vi "smartmeshIP get data packet.vi"(6 "use correction":bool=TRUE, 8 "error in":errorcluster, 10 "commandType":u8, 11 "data":string) -> (0 "error out":errorcluster, 2 "mote and link status":T2, 3 "Data Notifications":T3)   [LabVIEW 2017]
panel:
  out "network time":T1
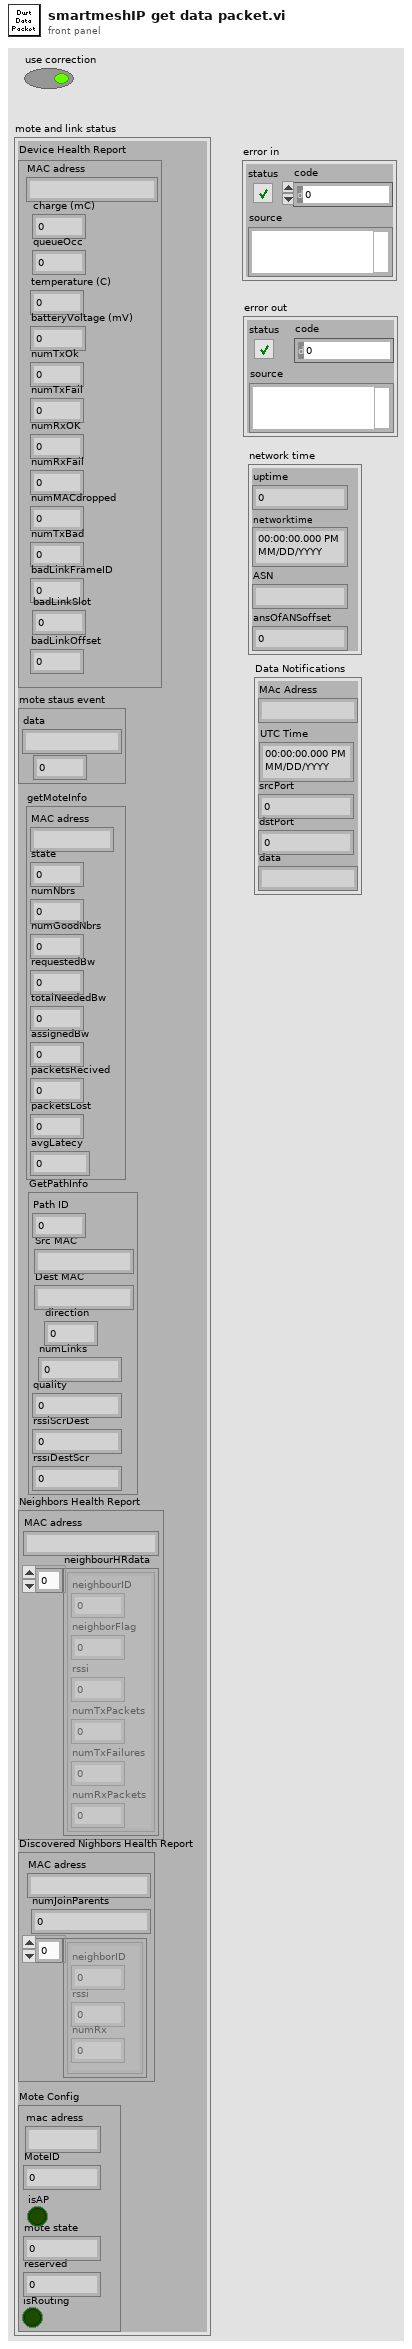
[diagram p1: front panel]
types:
  T1 = cluster{"uptime":u32, "networktime":timestamp, "ASN":string, "ansOfANSoffset":u16}
  T2 = cluster{"Device Health Report":cluster{"MAC adress":string, "charge (mC)":u32, "queueOcc":u8, "temperature (C)":i8, "batteryVoltage (mV)":u16, "numTxOk":u16, "numTxFail":u16, "numRxOK":u16, "numRxFail":u16, "numMACdropped":u8, "numTxBad":u8, "badLinkFrameID":u8, "badLinkSlot":u32, "badLinkOffset":u8}, "mote staus event":cluster{"data":string, u8}, "getMoteInfo":cluster{"MAC adress":string, "state":u8, "numNbrs":u8, "numGoodNbrs":u8, "requestedBw":u32, "totalNeededBw":u32, "assignedBw":u32, "packetsRecived":u32, "packetsLost":u32, "avgLatecy":u32}, "GetPathInfo":cluster{"Path ID":u8, "Src MAC":string, "Dest MAC":string, "direction":u8, "numLinks":u8, "quality":u8, "rssiScrDest":i8, "rssiDestScr":i8}, "Neighbors Health Report":cluster{"MAC adress":string, "neighbourHRdata":cluster{"neighbourID":u16, "neighborFlag":u8, "rssi":i8, "numTxPackets":u16, "numTxFailures":u16, "numRxPackets":u16}[]}, "Discovered Nighbors Health Report":cluster{"MAC adress":string, "numJoinParents":u8, cluster{"neighborID":u16, "rssi":i8, "numRx":u8}[]}, "Mote Config":cluster{"mac adress":string, "MoteID":u16, "isAP":bool, "mote state":u8, "reserved":u8, "isRouting":bool}}
  T3 = cluster{"MAc Adress":string, "UTC Time":timestamp, "srcPort":u16, "dstPort":u16, "data":string}
  T4 = cluster{"index":u32, "Dust Timestamp":timestamp, "data":string, "index":u16}
  T5 = cluster{"data":string, "Dust Timestamp":timestamp, u16, u16, "data":string}
  T6 = cluster{"data":string, u32, u8, i8, u16, u16, u16, u16, u16, u8, u8, u8, u32, u8}
  T7 = cluster{"data":string, cluster{u16, u8, i8, u16, u16, u16}[]}
  T8 = cluster{"data":string, u8, cluster{u16, i8, u8}[]}
  T9 = cluster{"(hi.lo)":u16, "data":string, "data":string, u8, u8, u8, i8, i8}
  T10 = cluster{u16, "data":string, "data":string, u8, u8, u8, i8, i8}
  T11 = cluster{"data":string, u8, u8, u8, u32, u32, u32, u32, u32, u32}
  T12 = cluster{cluster{"data":string, u32, u8, i8, u16, u16, u16, u16, u16, u8, u8, u8, u32, u8}, cluster{"data":string, i32}, cluster{"data":string, u8, u8, u8, u32, u32, u32, u32, u32, u32}, cluster{"(hi.lo)":u16, "data":string, "data":string, u8, u8, u8, i8, i8}, cluster{"data":string, cluster{u16, u8, i8, u16, u16, u16}[]}, cluster{"data":string, u8, cluster{u16, i8, u8}[]}, cluster{"data":string, u16, bool, u8, u8, bool}}
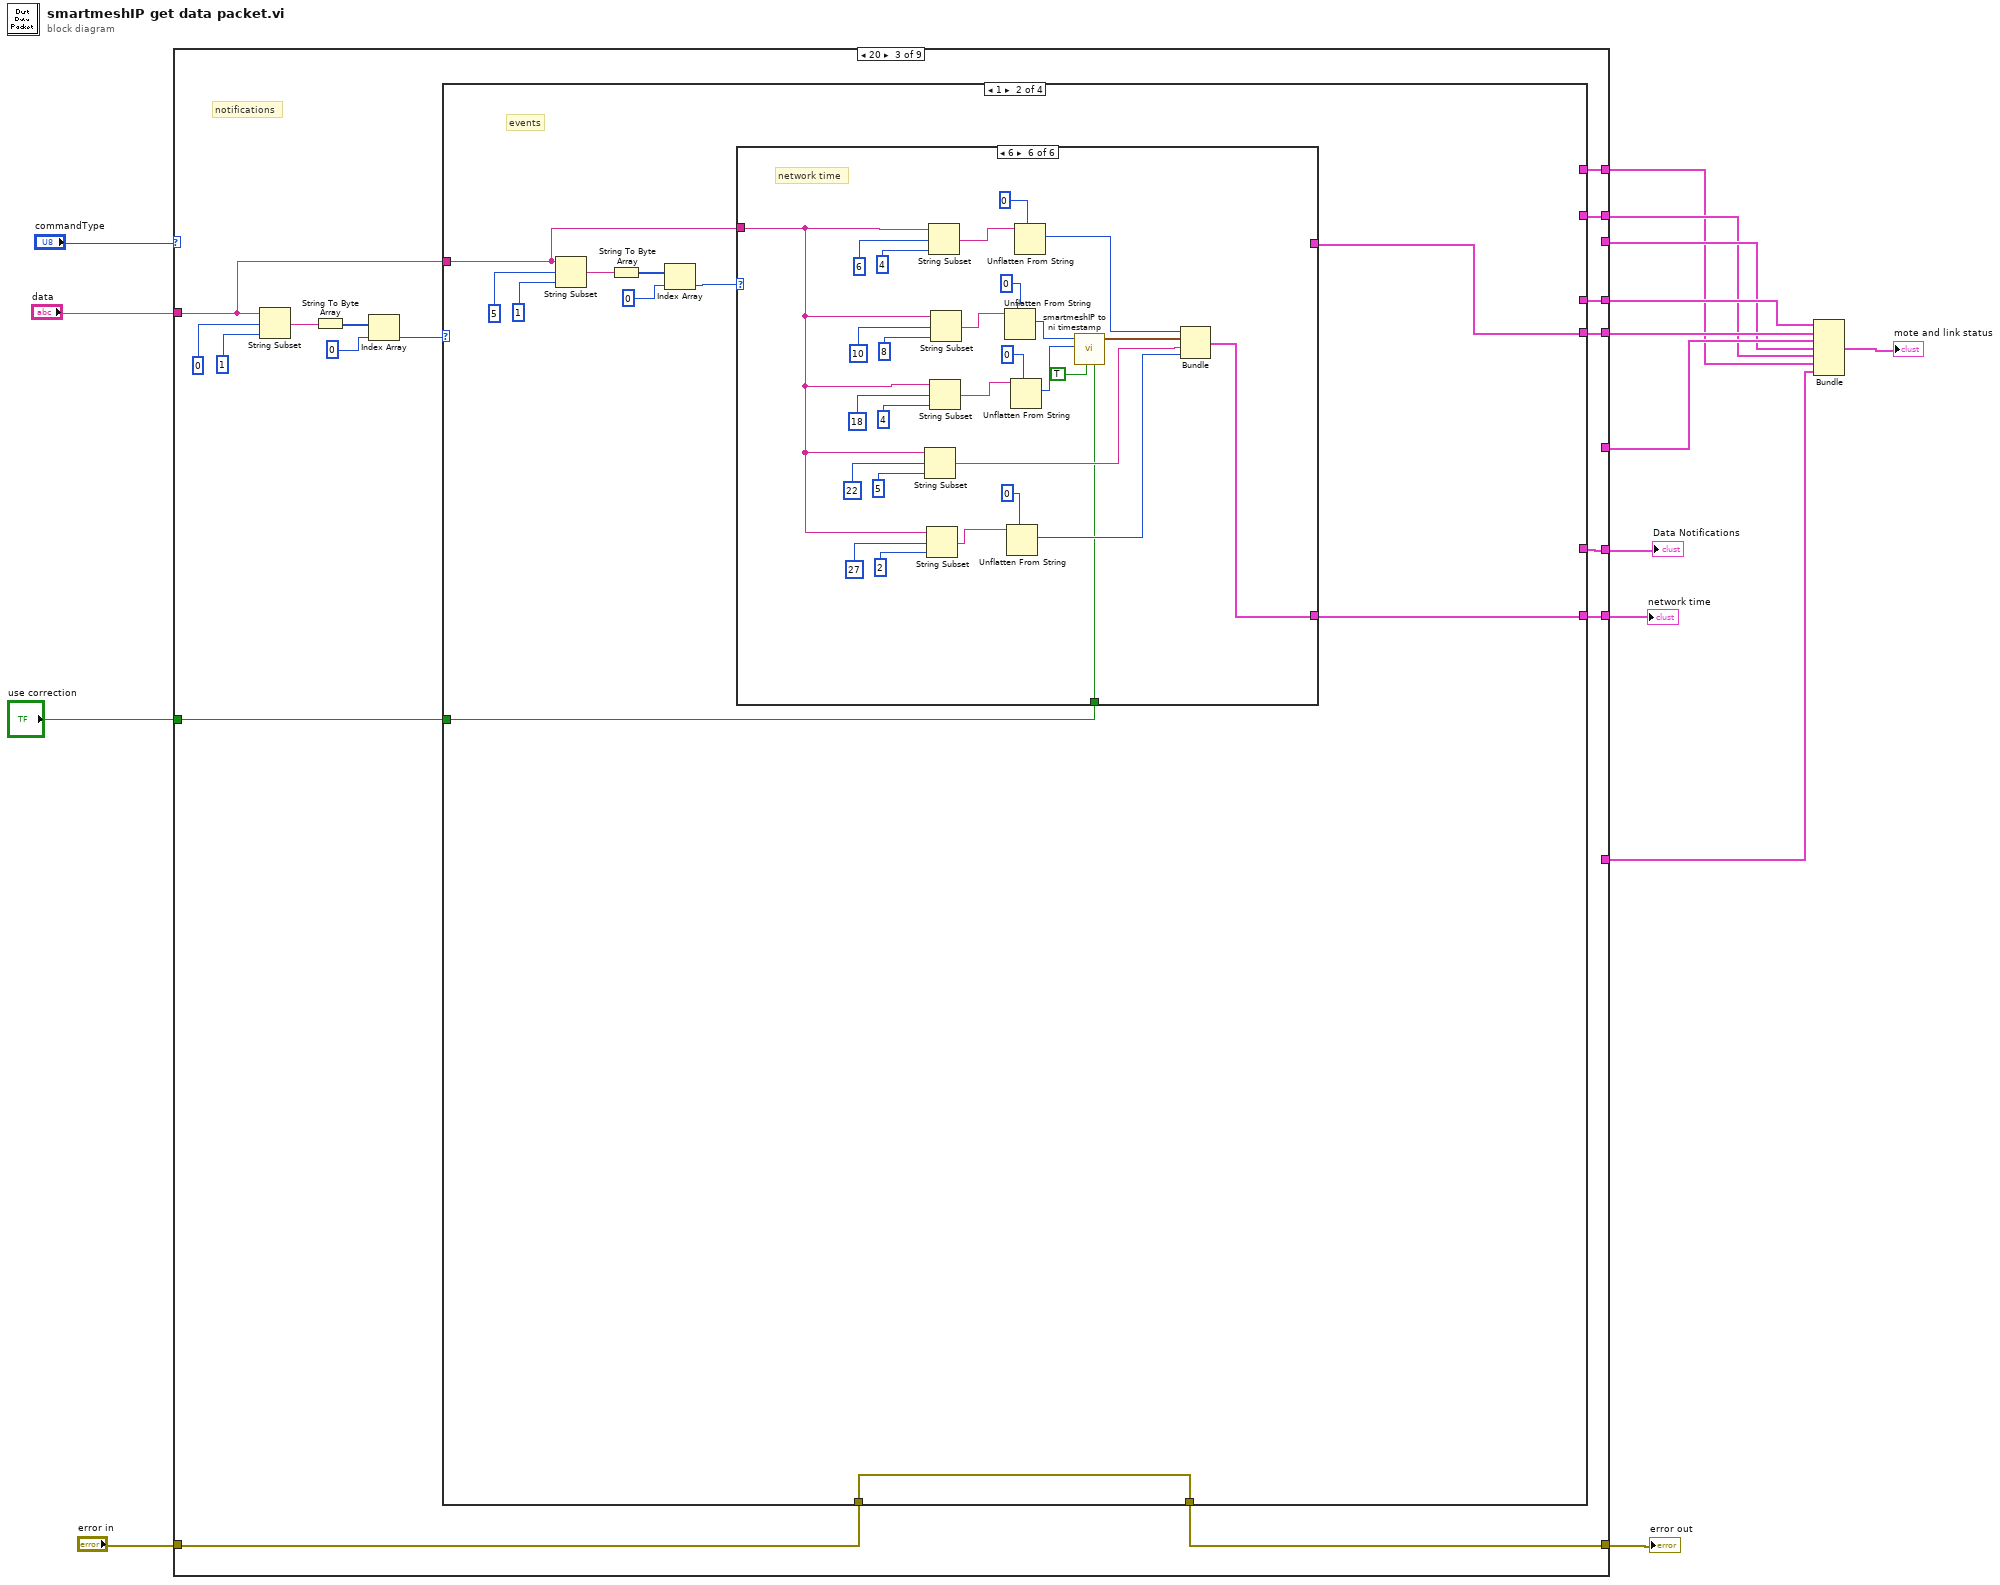
[diagram p0: block diagram]
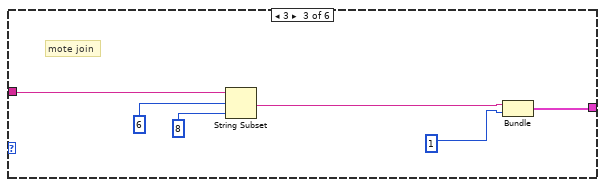
[diagram p7: hidden frame]
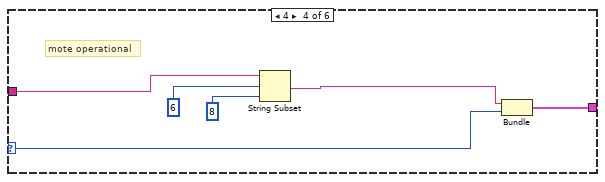
[diagram p8: hidden frame]
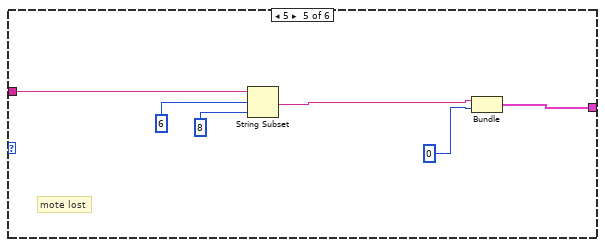
[diagram p9: hidden frame]
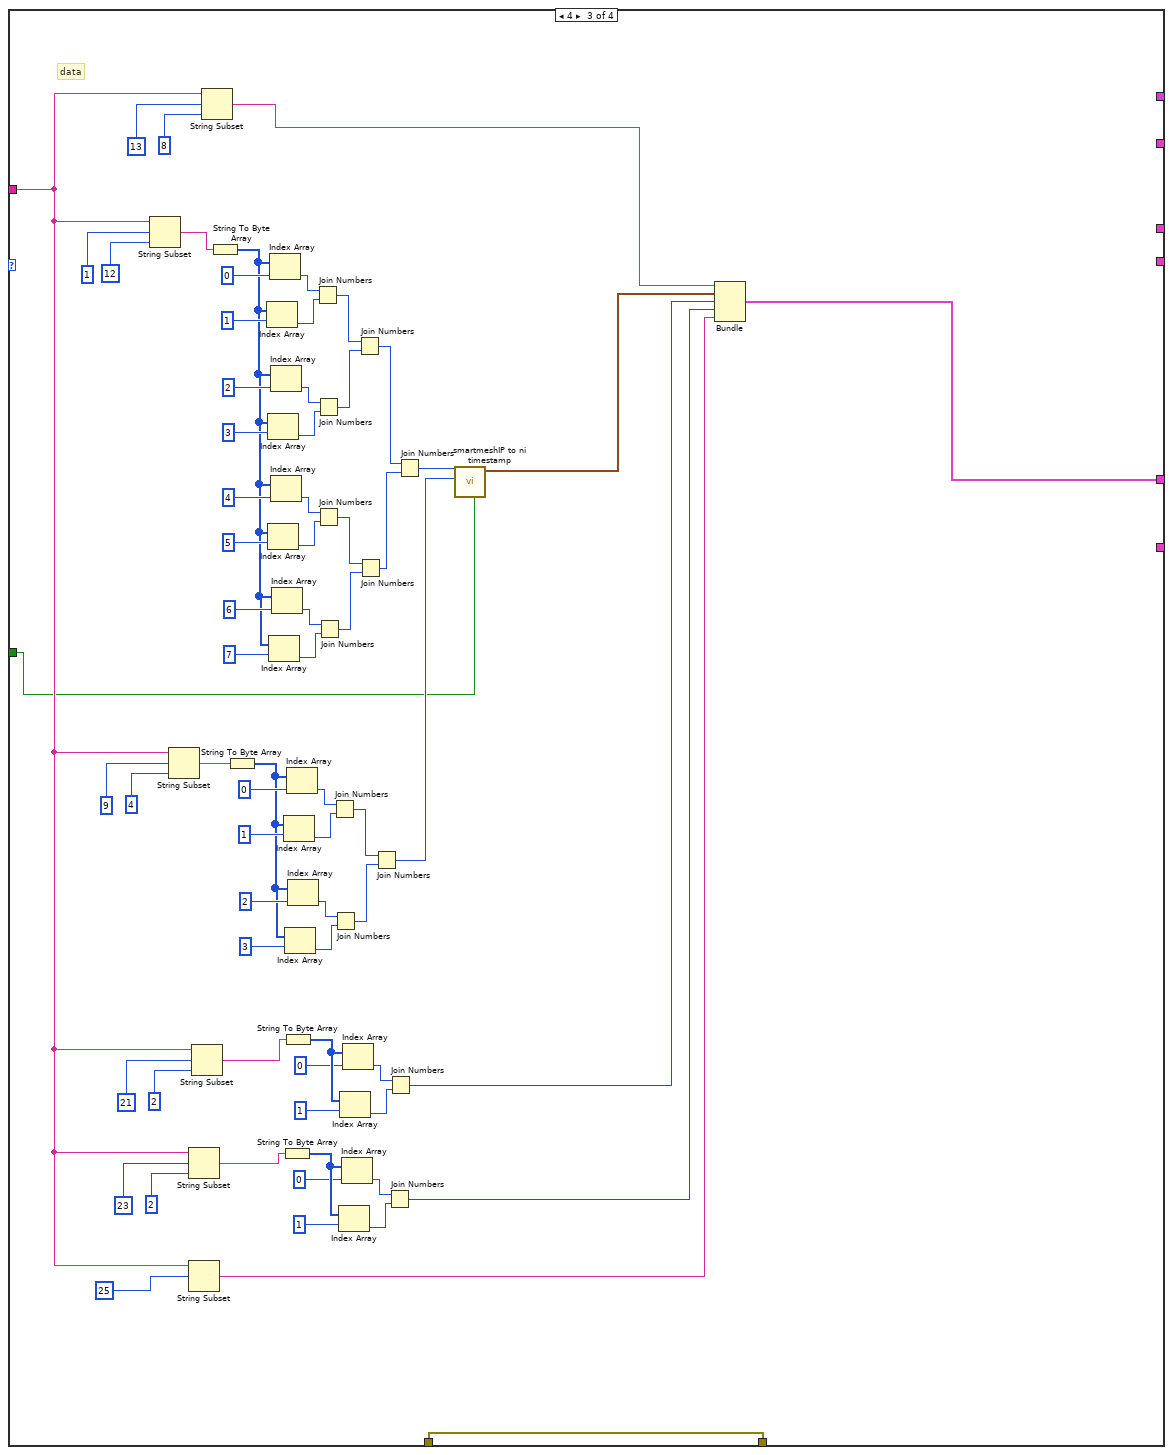
[diagram p10: hidden frame]
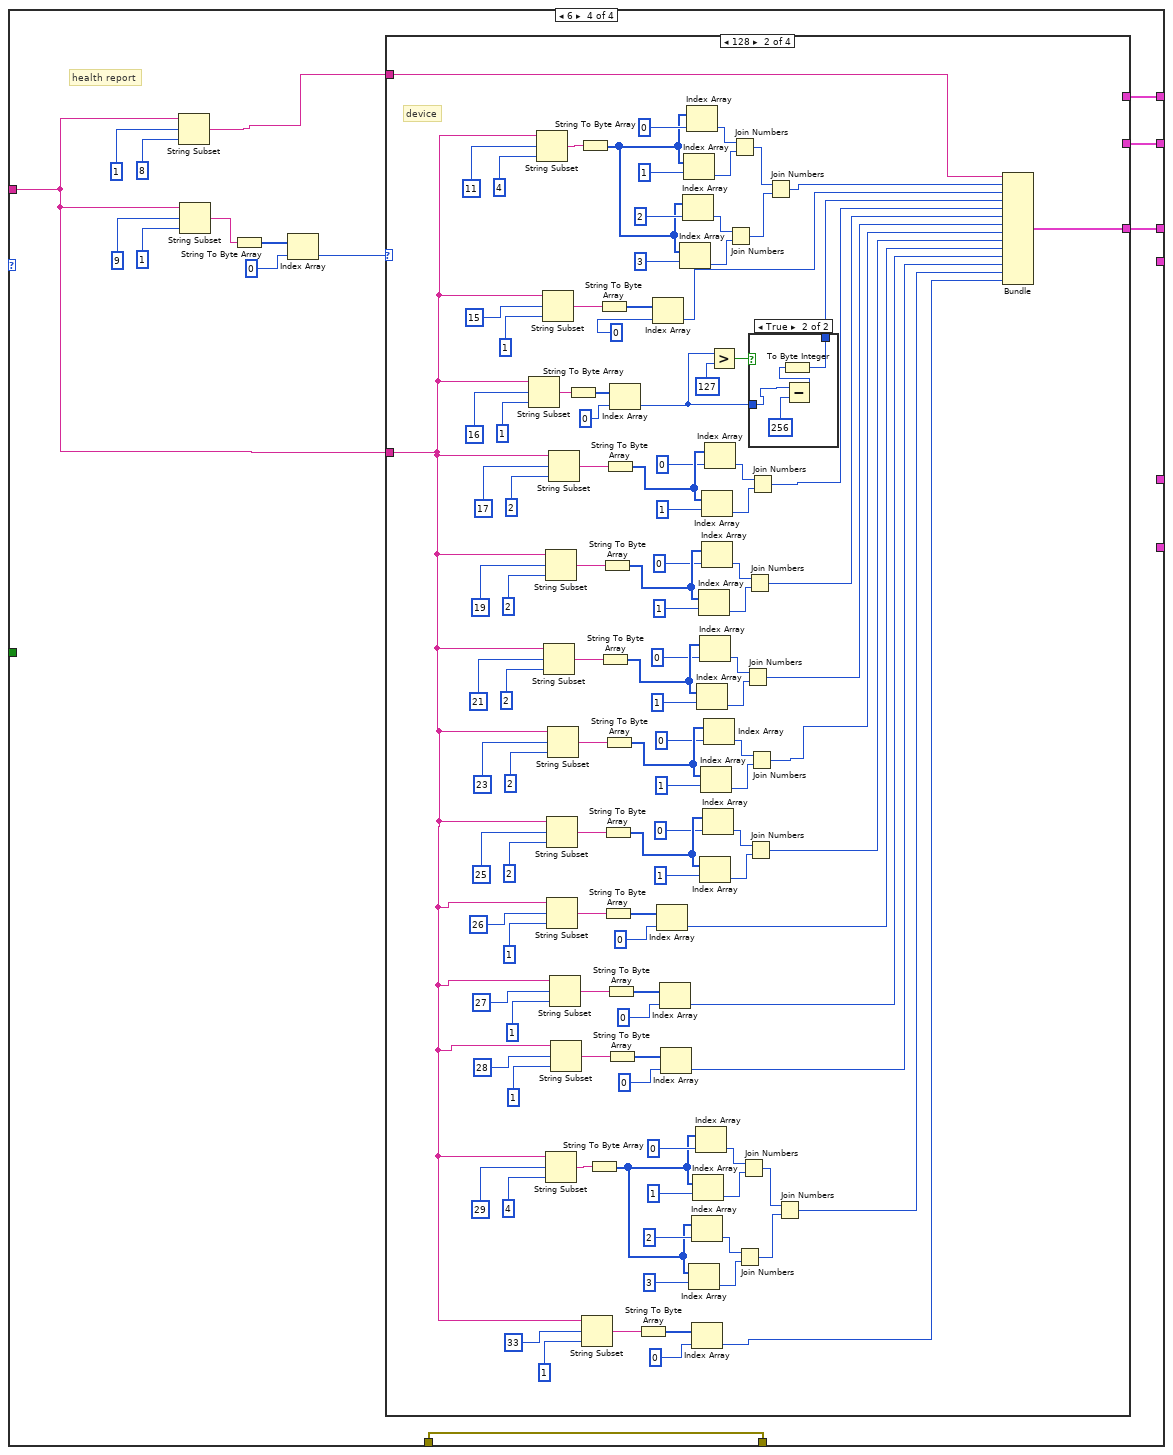
[diagram p11: hidden frame]
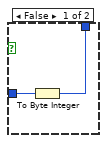
[diagram p13: hidden frame]
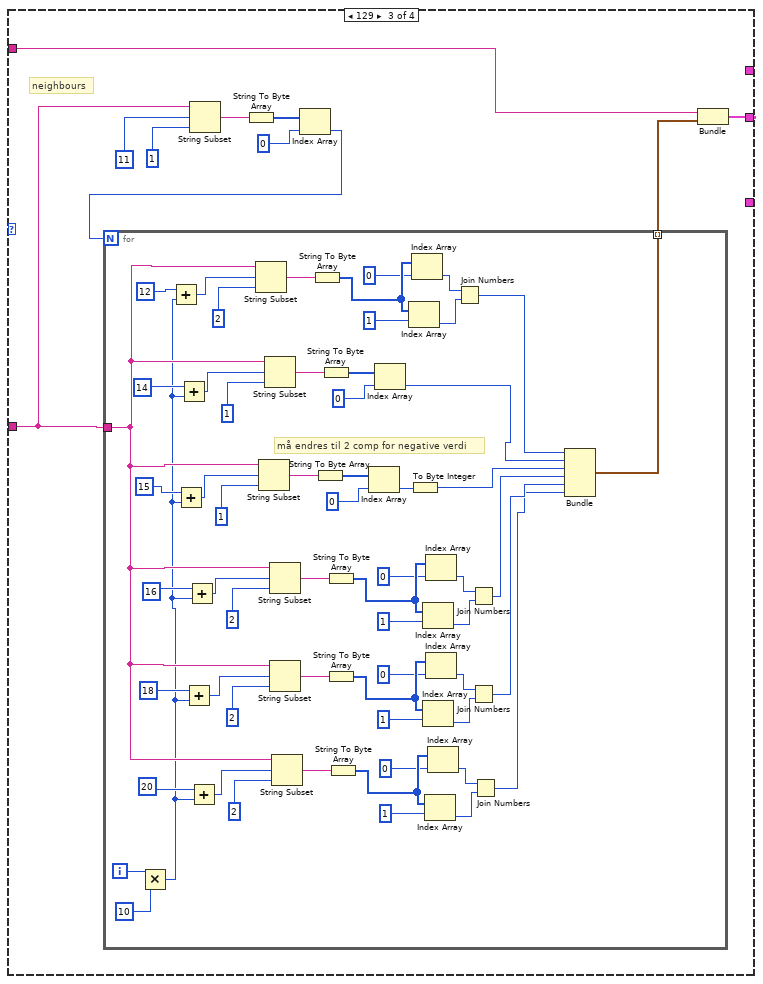
[diagram p14: hidden frame]
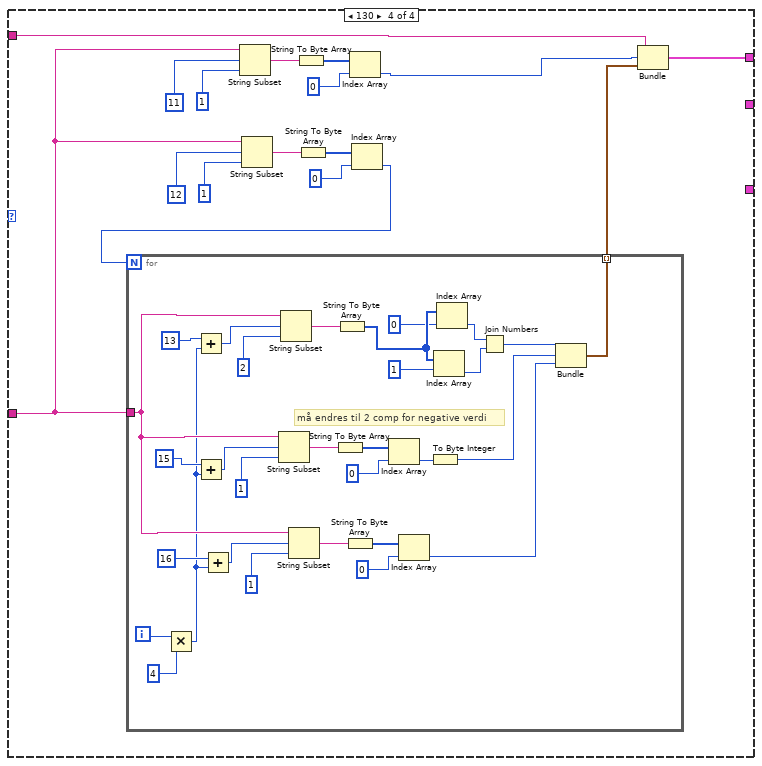
[diagram p15: hidden frame]
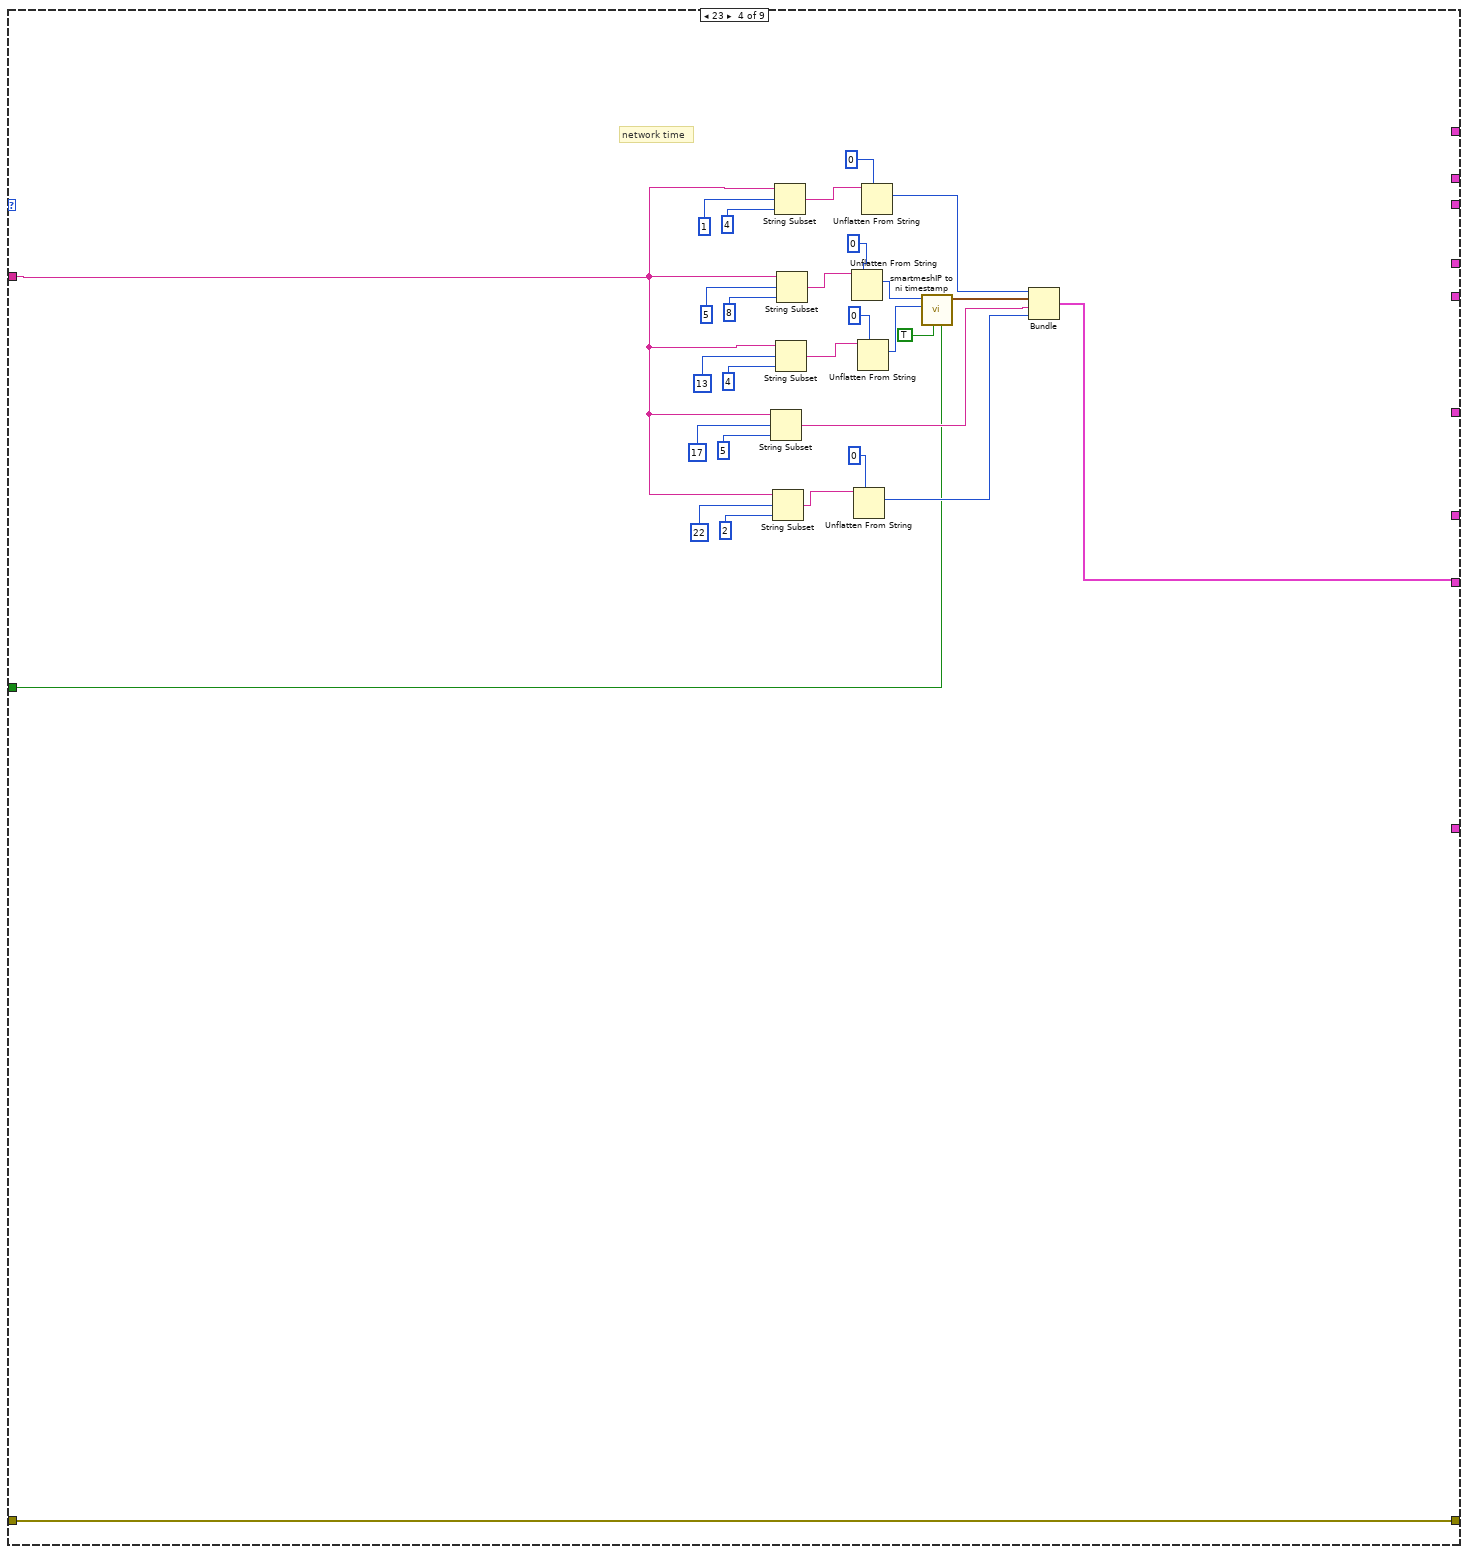
[diagram p16: hidden frame]
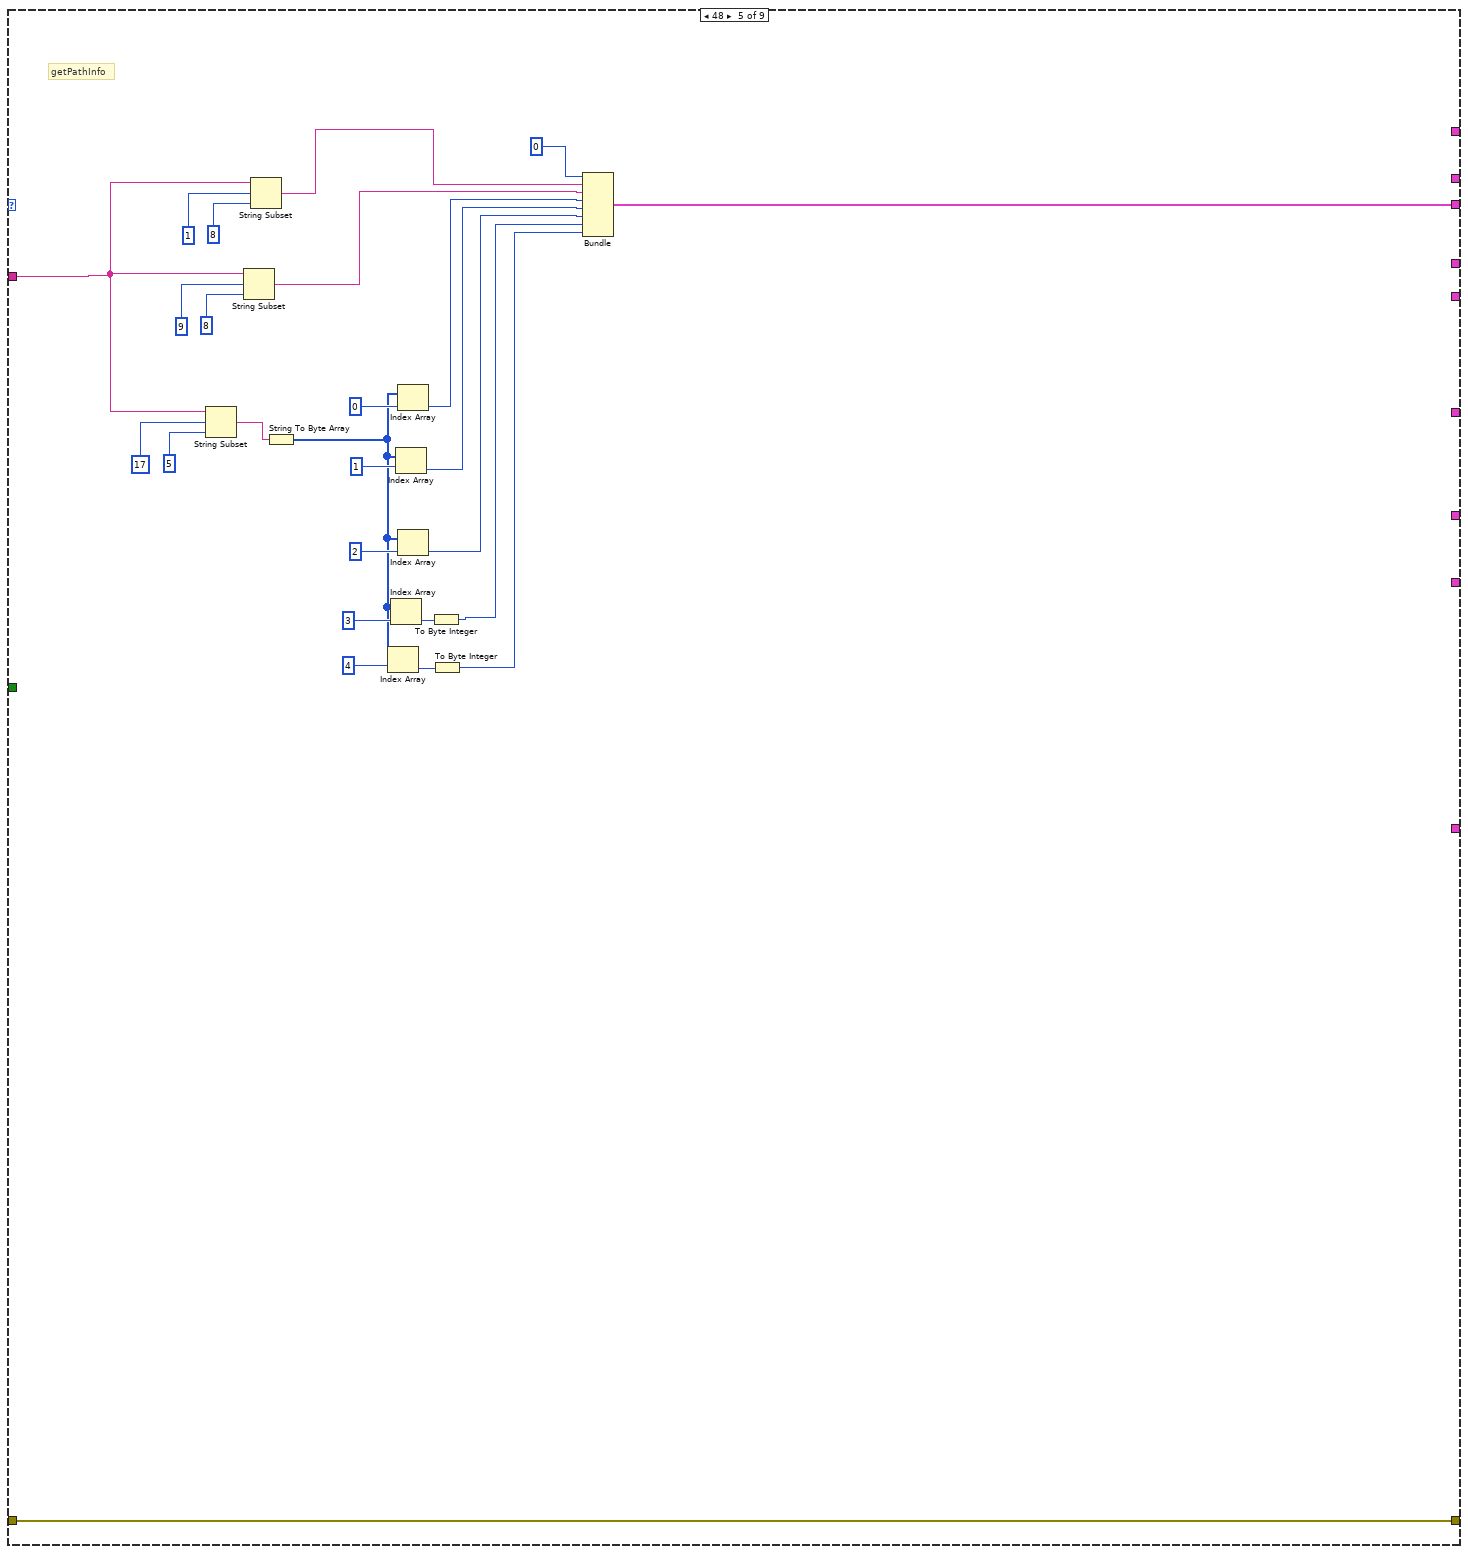
[diagram p17: hidden frame]
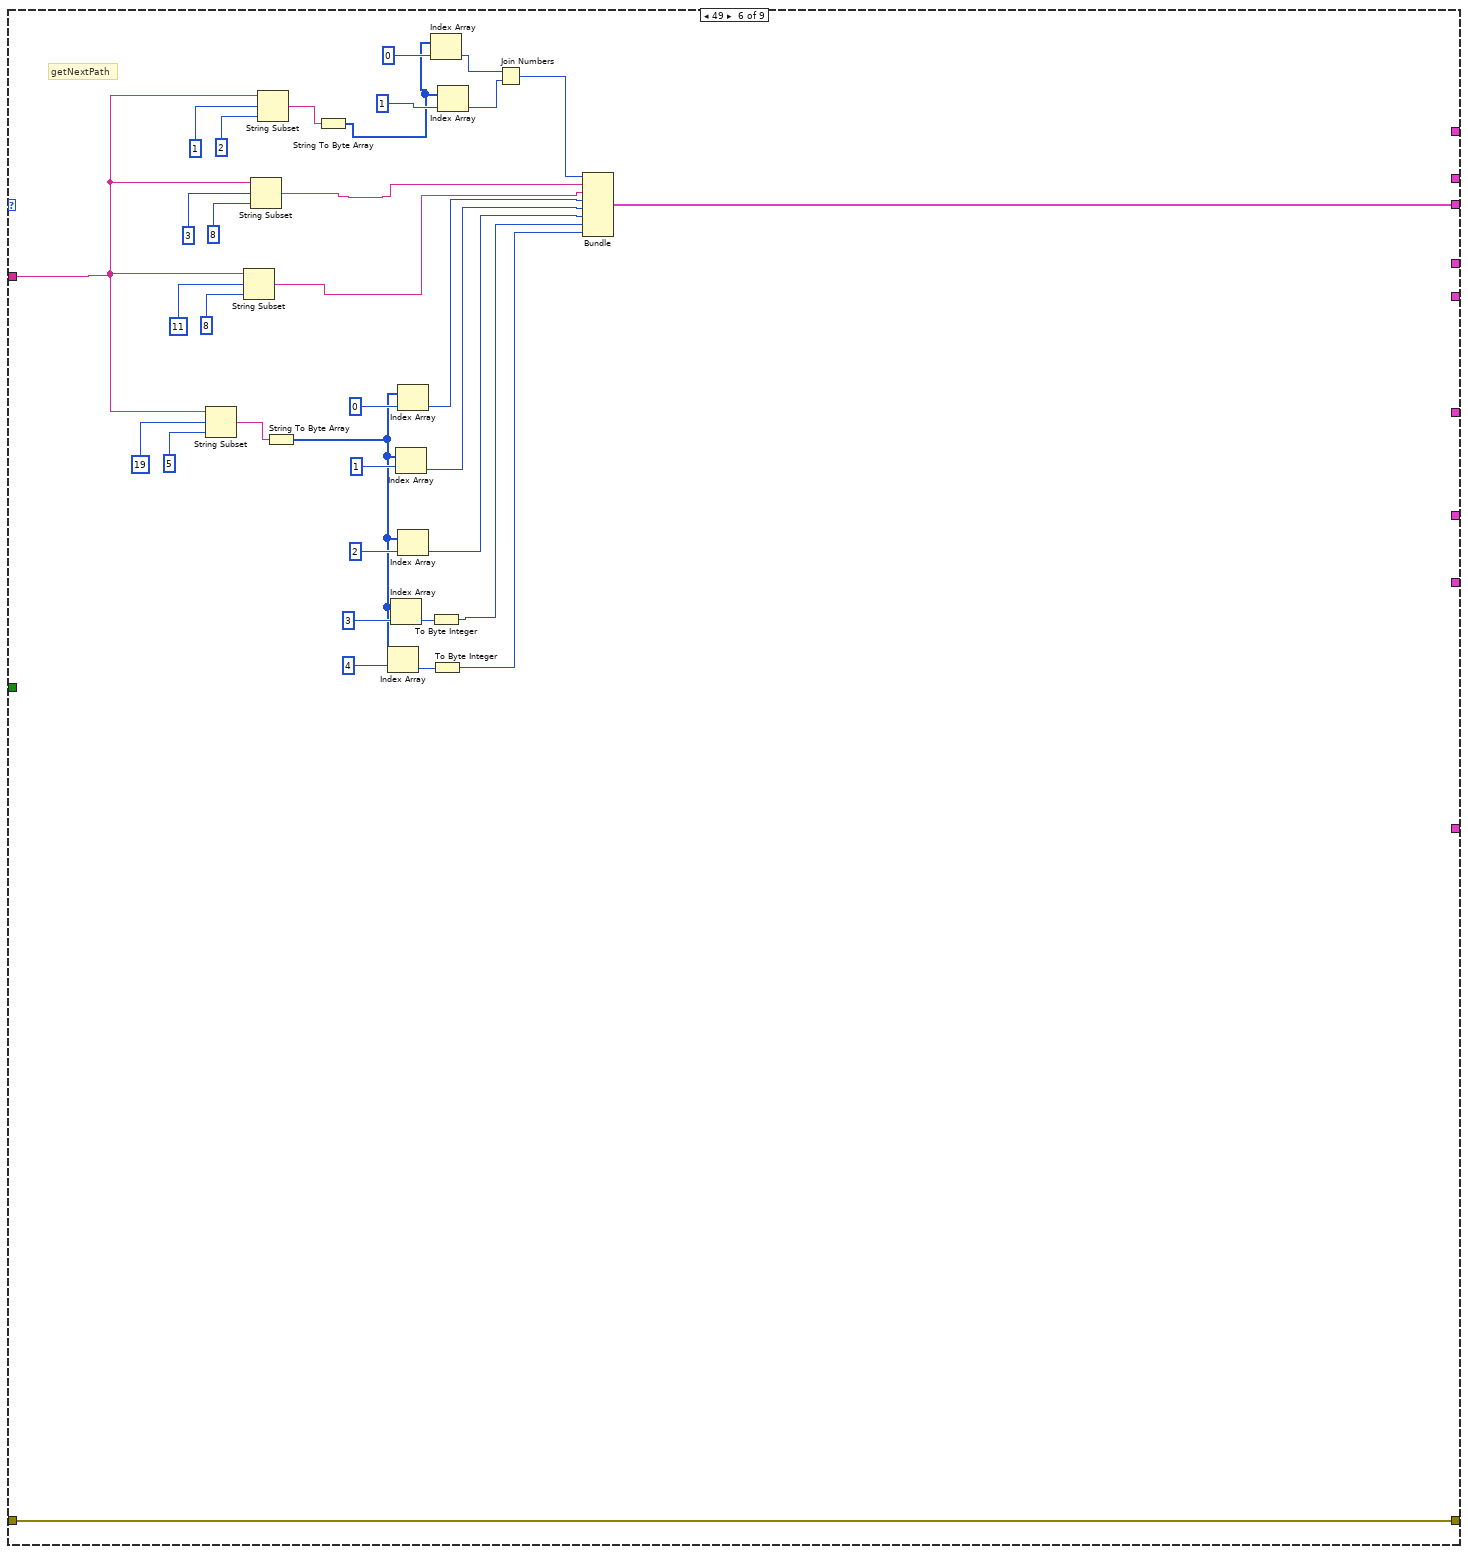
[diagram p18: hidden frame]
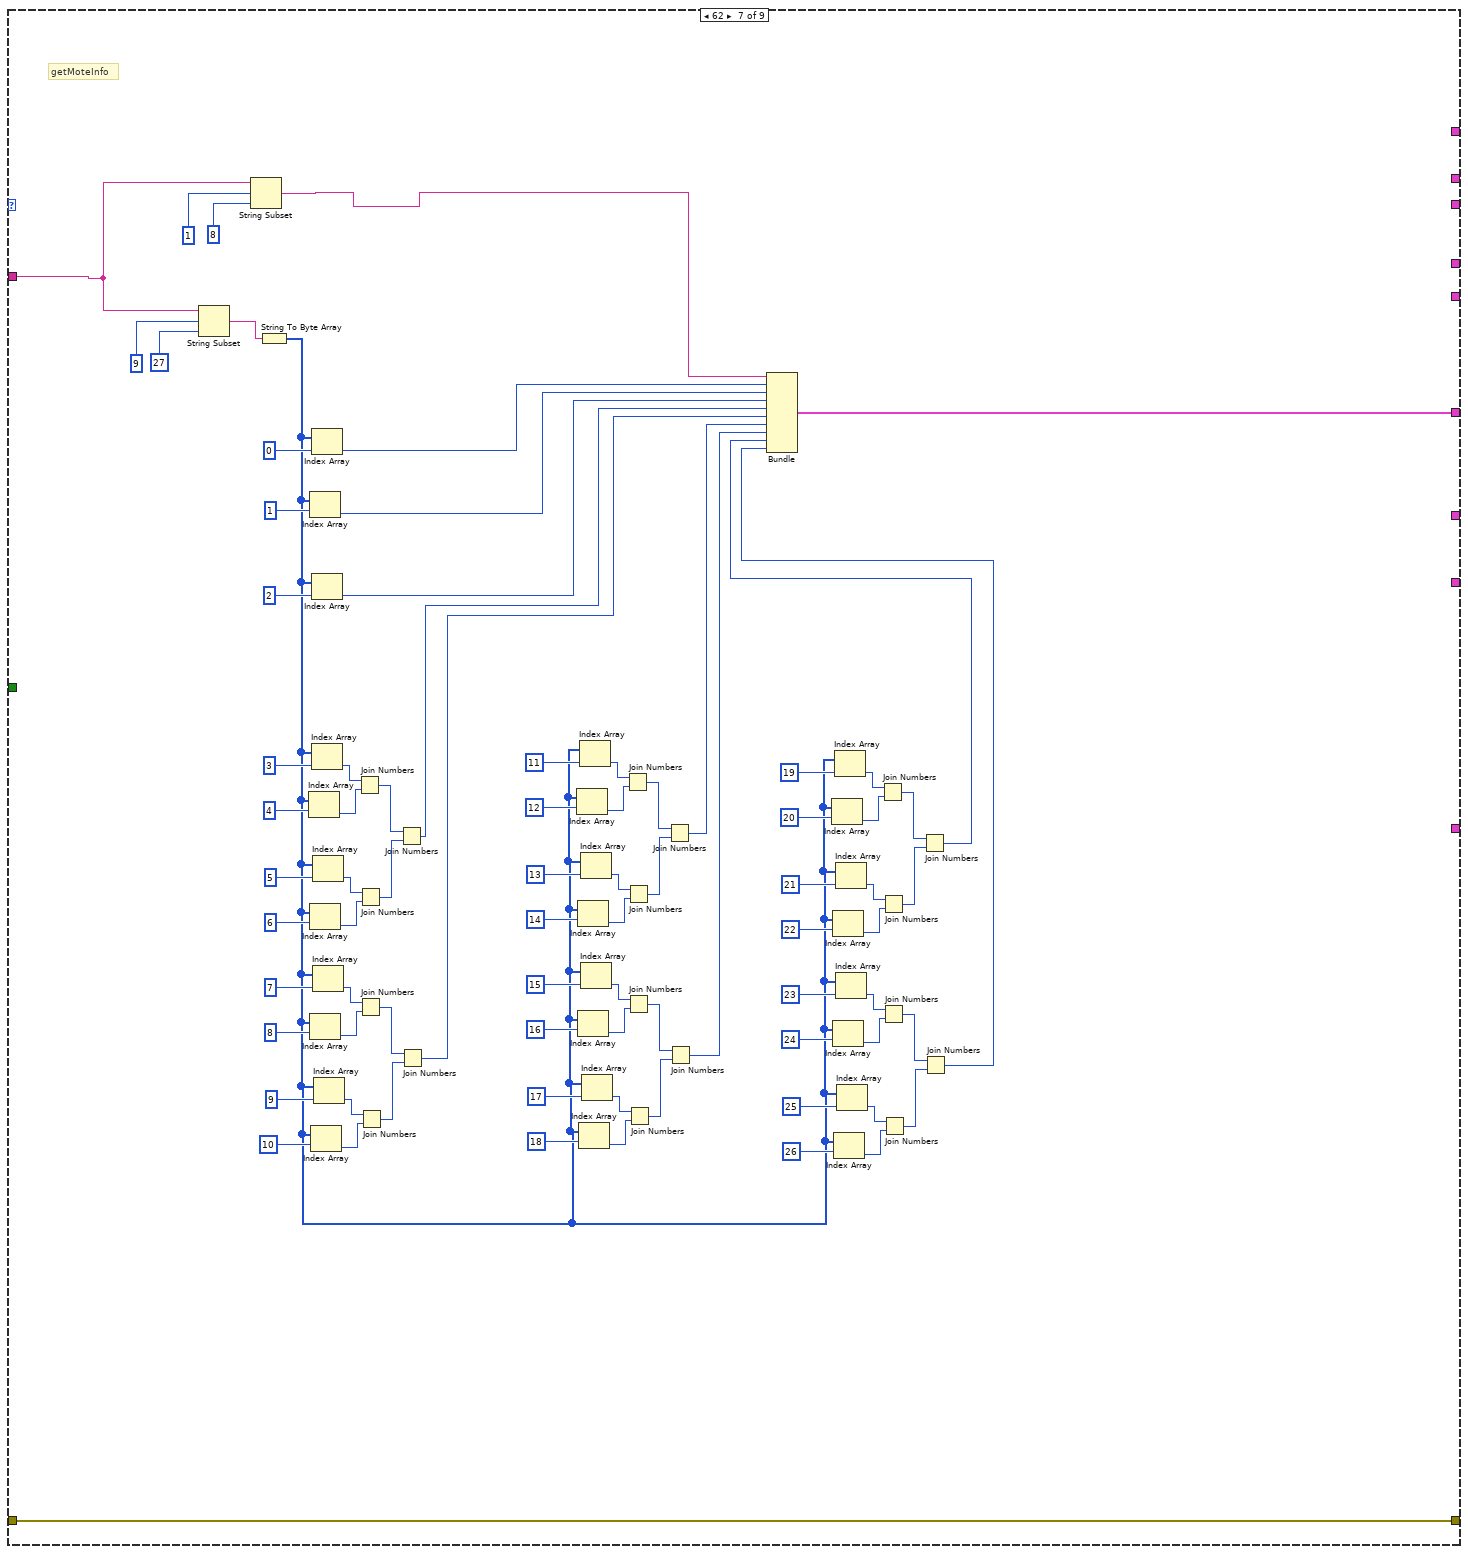
[diagram p19: hidden frame]
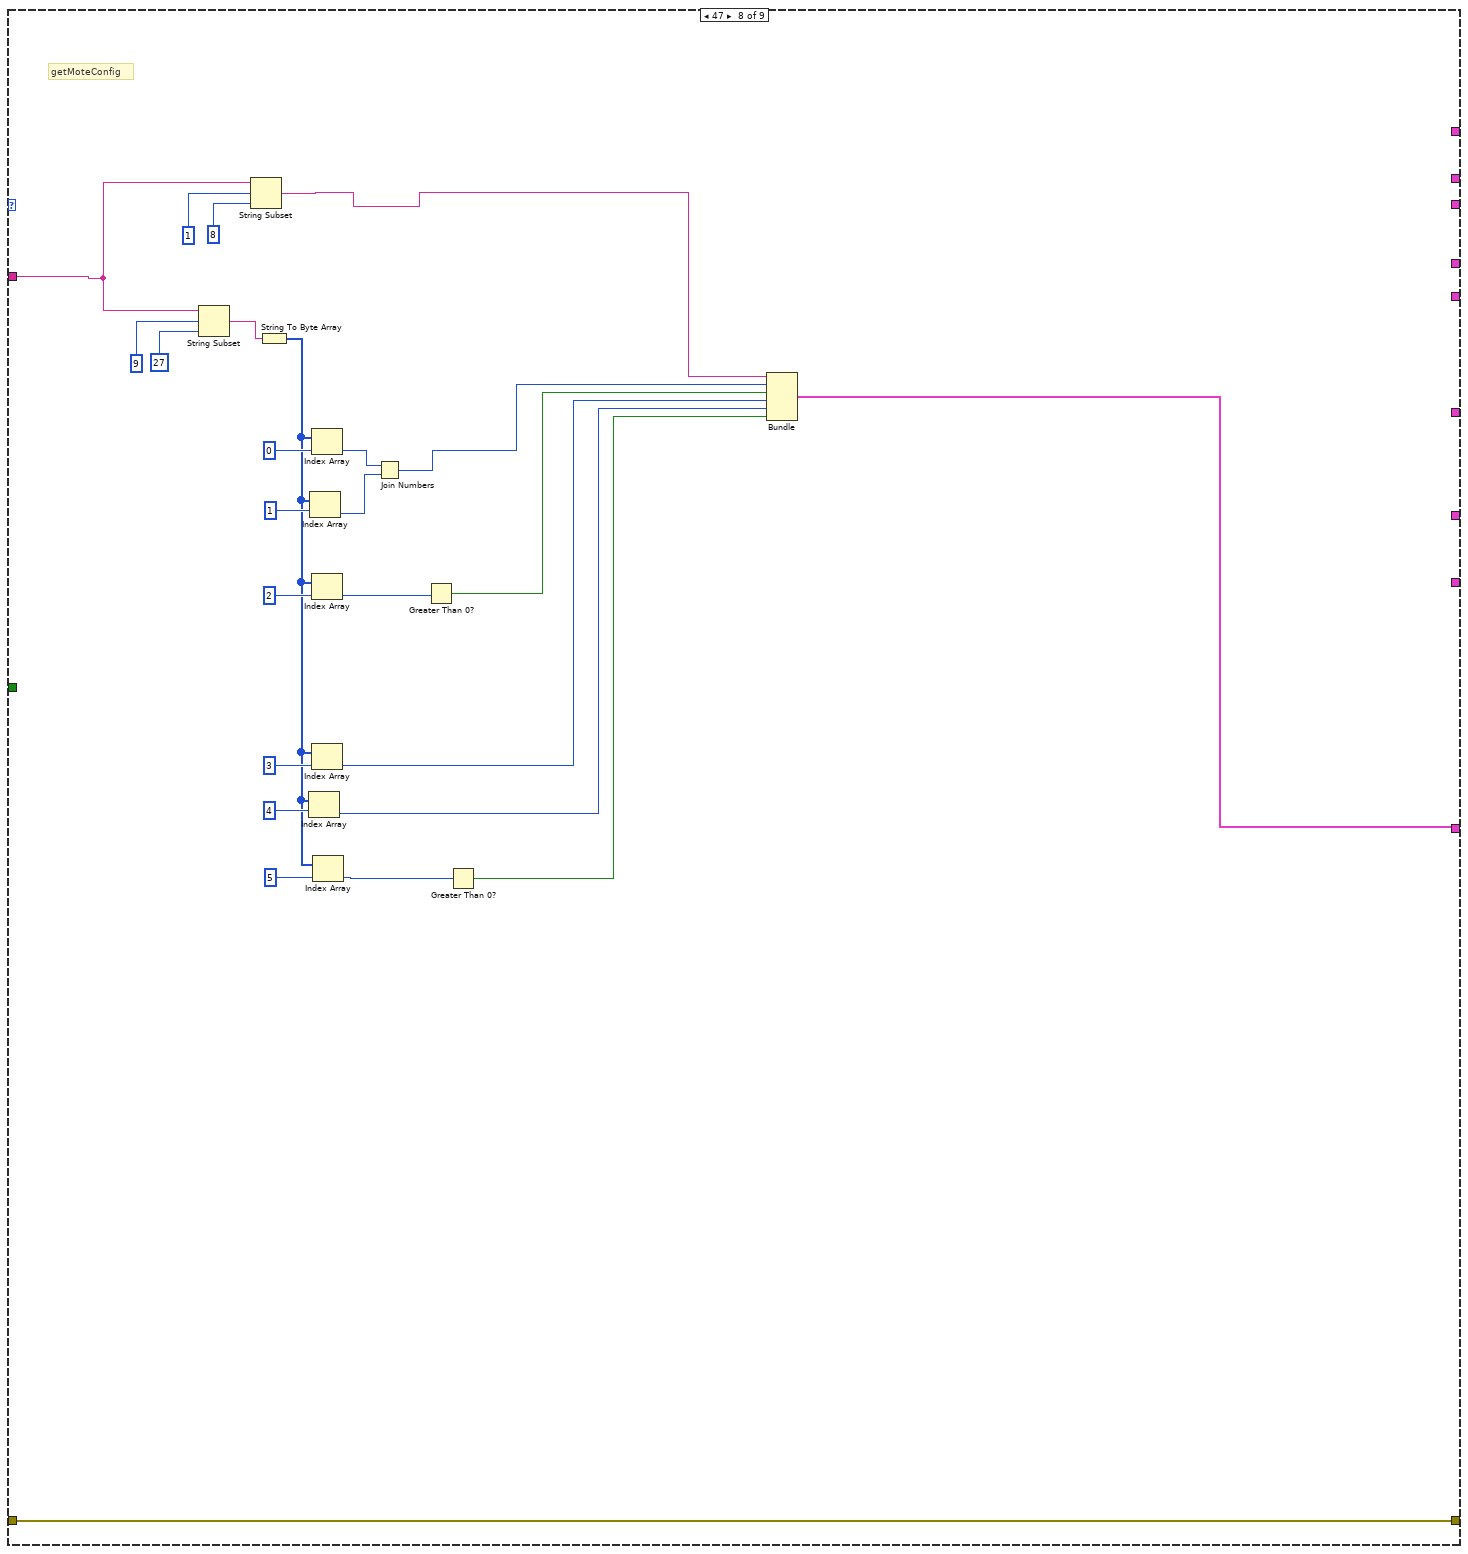
[diagram p20: hidden frame]
diagram:
  n1 = case shown="20" "commandType" {
    tunnel: "data" -> [_ _ w27 w418 w456 w487 w517 w599 w624]
    tunnel: [_ _ w26 _ _ _ _ _ _] -> w12
    tunnel: [_ _ w25 _ _ _ _ _ _] -> w8
    tunnel: [_ _ w24 _ _ _ _ _ _] -> w7
    tunnel: [_ _ w23 _ _ _ _ _ _] -> w13
    tunnel: [_ _ _ _ _ _ w506 _ _] -> w11
    tunnel: [_ _ _ _ w451 w483 _ _ _] -> w9
    tunnel: [_ _ w22 _ _ _ _ _ _] -> w10
    tunnel: [_ _ w21 w419 _ _ _ _ _] -> w5
    tunnel: [_ _ _ _ _ _ _ w587 w612] -> w4
    tunnel: [w16 w17 w19 w417 w444 w470 w504 w586 w611] -> w3
    tunnel: "error in" -> [w16 w17 w20 w417 w444 w470 w504 w586 w611]
    tunnel: "use correction" -> [_ _ w18 w415 _ _ _ _ _]
    frame 0, Default {
    }
    frame 3 {
    }
    frame 20 {
      # "notifications"
      n2 = String Subset(string=w27, offset (0)=0, length (rest)=1 ("length (rest)")) -> (substring=w31:string)
      n3 = String To Byte Array(string=w31) -> (unsigned byte array=w30:u8[])
      n4 = Index Array(array=w30, index=0) -> (element=w28:u8)
      n5 = case shown="1" w28 {
        tunnel: w27 -> [_ w38 w129 w167]
        tunnel: [_ _ _ w166] -> w26
        tunnel: [_ _ _ w165] -> w25
        tunnel: [_ _ _ w164] -> w24
        tunnel: [_ _ w137 _] -> w23
        tunnel: [_ w39 _ _] -> w22
        tunnel: [_ w37 _ _] -> w21
        tunnel: w20 -> [w34 w36 w93 w162]
        tunnel: [w34 w36 w93 w162] -> w19
        tunnel: w18 -> [_ w35 w92 _]
        frame 0, Default {
        }
        frame 1 {
          # "events"
          n6 = String Subset(string=w38, offset (0)=5, length (rest)=1 ("length (rest)")) -> (substring=w43:string)
          n7 = String To Byte Array(string=w43) -> (unsigned byte array=w42:u8[])
          n8 = Index Array(array=w42, index=0) -> (element=w40:u8)
          n9 = case shown="6" w40 {
            selector: w40 -> [_ _ _ w57 _ _]
            tunnel: w38 -> [_ _ w47 w53 w59 w81]
            tunnel: [_ _ w51 w56 w63 _] -> w39
            tunnel: [_ _ _ _ _ w66] -> w37
            tunnel: w35 -> [_ _ _ _ _ w65]
            frame 0, Default {
            }
            frame 1 {
            }
            frame 3 {
              # "mote join"
              n10 = String Subset(string=w47, offset (0)=6, length (rest)=8 ("length (rest)")) -> (substring=w46:string)
              n11 = Bundle("data"=w46, 1) -> (w51:cluster{"data":string, i32})  [unwired: 1 in]
            }
            frame 4 {
              # "mote operational"
              n12 = String Subset(string=w53, offset (0)=6, length (rest)=8 ("length (rest)")) -> (substring=w52:string)
              n13 = Bundle("data"=w52, w57) -> (w56:cluster{"data":string, u8})  [unwired: 1 in]
            }
            frame 5 {
              # "mote lost"
              n14 = String Subset(string=w59, offset (0)=6, length (rest)=8 ("length (rest)")) -> (substring=w58:string)
              n15 = Bundle("data"=w58, 0) -> (w63:cluster{"data":string, i32})  [unwired: 1 in]
            }
            frame 6 {
              # "network time"
              n16 = String Subset(string=w81, offset (0)=22, length (rest)=5 ("length (rest)")) -> (substring=w68:string)
              n17 = String Subset(string=w81, offset (0)=27, length (rest)=2 ("length (rest)")) -> (substring=w77:string)
              n18 = String Subset(string=w81, offset (0)=6, length (rest)=4 ("length (rest)")) -> (substring=w80:string)
              n19 = String Subset(string=w81, offset (0)=18, length (rest)=4 ("length (rest)")) -> (substring=w78:string)
              n20 = String Subset(string=w81, offset (0)=10, length (rest)=8 ("length (rest)")) -> (substring=w79:string)
              n21 = Unflatten From String(type=u64 0 ("index"), binary string=w79) -> (value=w76:u64)  [unwired: 3 in, 2 out]
              n22 = Unflatten From String(type=u16 0 ("index"), binary string=w77) -> (value=w67:u16)  [unwired: 3 in, 2 out]
              n23 = Unflatten From String(type=u32 0 ("index"), binary string=w78) -> (value=w75:u32)  [unwired: 3 in, 2 out]
              n24 = Unflatten From String(type=u32 0 ("index"), binary string=w80) -> (value=w70:u32)  [unwired: 3 in, 2 out]
              n25 = call "smartmeshIP to ni timestamp.vi"("use correction"=w65, "set corr due to mismatch in manager time"=TRUE, "microeconds"=w75, "seconds"=w76) -> ("Dust Timestamp"=w69:timestamp)  [unwired: 7 in]
              n26 = Bundle("index"=w70, "Dust Timestamp"=w69, "data"=w68, "index"=w67) -> (w66:T4)  [unwired: 1 in]
            }
          }
        }
        frame 4 {
          # "data"
          n27 = String Subset(string=w129, offset (0)=1, length (rest)=12 ("length (rest)")) -> (substring=w100:string)
          n28 = String Subset(string=w129, offset (0)=9, length (rest)=4 ("length (rest)")) -> (substring=w130:string)
          n29 = String Subset(string=w129, offset (0)=23, length (rest)=2 ("length (rest)")) -> (substring=w141:string)
          n30 = String Subset(string=w129, offset (0)=25) -> (substring=w138:string)  [unwired: 1 in]
          n31 = String Subset(string=w129, offset (0)=21, length (rest)=2 ("length (rest)")) -> (substring=w142:string)
          n32 = String Subset(string=w129, offset (0)=13, length (rest)=8 ("length (rest)")) -> (substring=w97:string)
          n33 = String To Byte Array(string=w100) -> (unsigned byte array=w101:u8[])
          n34 = String To Byte Array(string=w130) -> (unsigned byte array=w124:u8[])
          n35 = Index Array(array=w101, index=1) -> (element=w119:u8)
          n36 = Index Array(array=w101, index=3) -> (element=w115:u8)
          n37 = Index Array(array=w101, index=5) -> (element=w109:u8)
          n38 = Index Array(array=w101, index=7) -> (element=w105:u8)
          n39 = Index Array(array=w101, index=0) -> (element=w118:u8)
          n40 = Index Array(array=w101, index=2) -> (element=w114:u8)
          n41 = Index Array(array=w101, index=4) -> (element=w108:u8)
          n42 = Index Array(array=w101, index=6) -> (element=w104:u8)
          n43 = String To Byte Array(string=w141) -> (unsigned byte array=w146:u8[])
          n44 = String To Byte Array(string=w142) -> (unsigned byte array=w151:u8[])
          n45 = Index Array(array=w124, index=1) -> (element=w132:u8)
          n46 = Index Array(array=w124, index=3) -> (element=w126:u8)
          n47 = Index Array(array=w124, index=0) -> (element=w131:u8)
          n48 = Index Array(array=w124, index=2) -> (element=w125:u8)
          n49 = Join Numbers(hi=w118, lo=w119) -> ((hi.lo)=w112:u16)
          n50 = Join Numbers(hi=w114, lo=w115) -> ((hi.lo)=w113:u16)
          n51 = Join Numbers(hi=w108, lo=w109) -> ((hi.lo)=w102:u16)
          n52 = Join Numbers(hi=w104, lo=w105) -> ((hi.lo)=w103:u16)
          n53 = Join Numbers(hi=w131, lo=w132) -> ((hi.lo)=w122:u16)
          n54 = Join Numbers(hi=w125, lo=w126) -> ((hi.lo)=w123:u16)
          n55 = Index Array(array=w146, index=1) -> (element=w144:u8)
          n56 = Index Array(array=w151, index=1) -> (element=w149:u8)
          n57 = Index Array(array=w146, index=0) -> (element=w143:u8)
          n58 = Index Array(array=w151, index=0) -> (element=w148:u8)
          n59 = Join Numbers(hi=w112, lo=w113) -> ((hi.lo)=w98:u32)
          n60 = Join Numbers(hi=w102, lo=w103) -> ((hi.lo)=w99:u32)
          n61 = Join Numbers(hi=w122, lo=w123) -> ((hi.lo)=w95:u32)
          n62 = Join Numbers(hi=w143, lo=w144) -> ((hi.lo)=w139:u16)
          n63 = Join Numbers(hi=w148, lo=w149) -> ((hi.lo)=w140:u16)
          n64 = Join Numbers(hi=w98, lo=w99) -> ((hi.lo)=w96:u64)
          n65 = call "smartmeshIP to ni timestamp.vi"("use correction"=w92, "microeconds"=w95, "seconds"=w96) -> ("Dust Timestamp"=w94:timestamp)  [unwired: 8 in]
          n66 = Bundle("data"=w97, "Dust Timestamp"=w94, w140, w139, "data"=w138) -> (w137:T5)  [unwired: 1 in]
        }
        frame 6 {
          # "health report"
          n67 = String Subset(string=w167, offset (0)=1, length (rest)=8 ("length (rest)")) -> (substring=w163:string)
          n68 = String Subset(string=w167, offset (0)=9, length (rest)=1 ("length (rest)")) -> (substring=w169:string)
          n69 = String To Byte Array(string=w169) -> (unsigned byte array=w171:u8[])
          n70 = Index Array(array=w171, index=0) -> (element=w168:u8)
          n71 = case shown="128" w168 {
            tunnel: w167 -> [_ w196 w303 w373]
            tunnel: w163 -> [_ w195 w302 w372]
            tunnel: [_ w182 _ _] -> w166
            tunnel: [_ _ w299 _] -> w165
            tunnel: [_ _ _ w369] -> w164
            frame 0, Default {
            }
            frame 128 {
              # "device"
              n72 = String Subset(string=w196, offset (0)=16, length (rest)=1 ("length (rest)")) -> (substring=w180:string)
              n73 = String Subset(string=w196, offset (0)=11, length (rest)=4 ("length (rest)")) -> (substring=w270:string)
              n74 = String Subset(string=w196, offset (0)=15, length (rest)=1 ("length (rest)")) -> (substring=w181:string)
              n75 = String Subset(string=w196, offset (0)=21, length (rest)=2 ("length (rest)")) -> (substring=w247:string)
              n76 = String Subset(string=w196, offset (0)=19, length (rest)=2 ("length (rest)")) -> (substring=w255:string)
              n77 = String Subset(string=w196, offset (0)=29, length (rest)=4 ("length (rest)")) -> (substring=w209:string)
              n78 = String Subset(string=w196, offset (0)=25, length (rest)=2 ("length (rest)")) -> (substring=w231:string)
              n79 = String Subset(string=w196, offset (0)=26, length (rest)=1 ("length (rest)")) -> (substring=w228:string)
              n80 = String Subset(string=w196, offset (0)=23, length (rest)=2 ("length (rest)")) -> (substring=w239:string)
              n81 = String Subset(string=w196, offset (0)=17, length (rest)=2 ("length (rest)")) -> (substring=w282:string)
              n82 = String Subset(string=w196, offset (0)=27, length (rest)=1 ("length (rest)")) -> (substring=w223:string)
              n83 = String Subset(string=w196, offset (0)=28, length (rest)=1 ("length (rest)")) -> (substring=w218:string)
              n84 = String To Byte Array(string=w180) -> (unsigned byte array=w281:u8[])
              n85 = String To Byte Array(string=w270) -> (unsigned byte array=w265:u8[])
              n86 = String Subset(string=w196, offset (0)=33, length (rest)=1 ("length (rest)")) -> (substring=w199:string)
              n87 = String To Byte Array(string=w209) -> (unsigned byte array=w204:u8[])
              n88 = String To Byte Array(string=w181) -> (unsigned byte array=w278:u8[])
              n89 = String To Byte Array(string=w247) -> (unsigned byte array=w251:u8[])
              n90 = String To Byte Array(string=w255) -> (unsigned byte array=w259:u8[])
              n91 = String To Byte Array(string=w231) -> (unsigned byte array=w235:u8[])
              n92 = String To Byte Array(string=w228) -> (unsigned byte array=w227:u8[])
              n93 = String To Byte Array(string=w239) -> (unsigned byte array=w243:u8[])
              n94 = String To Byte Array(string=w282) -> (unsigned byte array=w286:u8[])
              n95 = String To Byte Array(string=w223) -> (unsigned byte array=w222:u8[])
              n96 = String To Byte Array(string=w218) -> (unsigned byte array=w217:u8[])
              n97 = Index Array(array=w281, index=0) -> (element=w176:u8)
              n98 = String To Byte Array(string=w199) -> (unsigned byte array=w198:u8[])
              n99 = Index Array(array=w278, index=0) -> (element=w193:u8)
              n100 = Index Array(array=w227, index=0) -> (element=w187:u8)
              n101 = Index Array(array=w222, index=0) -> (element=w186:u8)
              n102 = Index Array(array=w217, index=0) -> (element=w185:u8)
              n103 = Index Array(array=w265, index=3) -> (element=w267:u8)
              n104 = Index Array(array=w265, index=2) -> (element=w266:u8)
              n105 = Index Array(array=w265, index=1) -> (element=w272:u8)
              n106 = Index Array(array=w265, index=0) -> (element=w271:u8)
              n107 = Index Array(array=w204, index=3) -> (element=w206:u8)
              n108 = Index Array(array=w204, index=2) -> (element=w205:u8)
              n109 = Index Array(array=w198, index=0) -> (element=w183:u8)
              n110 = Index Array(array=w204, index=1) -> (element=w211:u8)
              n111 = Index Array(array=w204, index=0) -> (element=w210:u8)
              n112 = Index Array(array=w251, index=1) -> (element=w249:u8)
              n113 = Index Array(array=w259, index=1) -> (element=w257:u8)
              n114 = Index Array(array=w251, index=0) -> (element=w248:u8)
              n115 = Index Array(array=w235, index=1) -> (element=w233:u8)
              n116 = Index Array(array=w243, index=1) -> (element=w241:u8)
              n117 = Index Array(array=w286, index=1) -> (element=w284:u8)
              n118 = Index Array(array=w259, index=0) -> (element=w256:u8)
              n119 = Index Array(array=w235, index=0) -> (element=w232:u8)
              n120 = Index Array(array=w243, index=0) -> (element=w240:u8)
              n121 = Index Array(array=w286, index=0) -> (element=w283:u8)
              n122 = Greater?(x=w176, y=u8 127) -> (0:w178:bool)
              n123 = Join Numbers(hi=w266, lo=w267) -> ((hi.lo)=w263:u16)
              n124 = Join Numbers(hi=w271, lo=w272) -> ((hi.lo)=w264:u16)
              n125 = Join Numbers(hi=w205, lo=w206) -> ((hi.lo)=w202:u16)
              n126 = Join Numbers(hi=w210, lo=w211) -> ((hi.lo)=w203:u16)
              n127 = Join Numbers(hi=w248, lo=w249) -> ((hi.lo)=w190:u16)
              n128 = Join Numbers(hi=w256, lo=w257) -> ((hi.lo)=w191:u16)
              n129 = Join Numbers(hi=w232, lo=w233) -> ((hi.lo)=w188:u16)
              n130 = Join Numbers(hi=w240, lo=w241) -> ((hi.lo)=w189:u16)
              n131 = Join Numbers(hi=w283, lo=w284) -> ((hi.lo)=w192:u16)
              n132 = case shown="True" w178 {
                tunnel: w176 -> [w294 w296]
                tunnel: [w293 w298] -> w177
                frame False {
                  n133 = To Byte Integer(number=w294) -> (8bit integer=w293:i8)
                }
                frame True {
                  n134 = Subtract(x=w296, y=u16 256) -> (x-y=w297:u16)
                  n135 = To Byte Integer(number=w297) -> (8bit integer=w298:i8)
                }
              }
              n136 = Join Numbers(hi=w264, lo=w263) -> ((hi.lo)=w194:u32)
              n137 = Join Numbers(hi=w203, lo=w202) -> ((hi.lo)=w184:u32)
              n138 = Bundle("data"=w195, w194, w193, w177, w192, w191, w190, w189, w188, w187, w186, w185, w184, w183) -> (w182:T6)  [unwired: 1 in]
            }
            frame 129 {
              # "neighbours"
              n139 = String Subset(string=w303, offset (0)=11, length (rest)=1 ("length (rest)")) -> (substring=w306:string)
              n140 = String To Byte Array(string=w306) -> (unsigned byte array=w305:u8[])
              n141 = Index Array(array=w305, index=0) -> (element=w301:u8)
              n142 = for {
                N: w301 -> [_]
                tunnel: w303 -> [w331]
                tunnel: [w309] -> w300 mode=indexing
                i -> [w330]
                # "må endres til 2 comp for negative verdi"
                n143 = Multiply(x=w330, y=10) -> (x*y=w316:i32)
                n144 = Add(x=12 ("offset (0)"), y=w316) -> (x+y=w328:i32)
                n145 = Add(x=15 ("offset (0)"), y=w316) -> (x+y=w324:i32)
                n146 = Add(x=14 ("offset (0)"), y=w316) -> (x+y=w326:i32)
                n147 = Add(x=18 ("offset (0)"), y=w316) -> (x+y=w320:i32)
                n148 = Add(x=16 ("offset (0)"), y=w316) -> (x+y=w321:i32)
                n149 = Add(x=20 ("offset (0)"), y=w316) -> (x+y=w318:i32)
                n150 = String Subset(string=w331, offset (0)=w328, length (rest)=2 ("length (rest)")) -> (substring=w362:string)
                n151 = String Subset(string=w331, offset (0)=w324, length (rest)=1 ("length (rest)")) -> (substring=w334:string)
                n152 = String Subset(string=w331, offset (0)=w326, length (rest)=1 ("length (rest)")) -> (substring=w339:string)
                n153 = String Subset(string=w331, offset (0)=w321, length (rest)=2 ("length (rest)")) -> (substring=w355:string)
                n154 = String Subset(string=w331, offset (0)=w320, length (rest)=2 ("length (rest)")) -> (substring=w348:string)
                n155 = String Subset(string=w331, offset (0)=w318, length (rest)=2 ("length (rest)")) -> (substring=w341:string)
                n156 = String To Byte Array(string=w362) -> (unsigned byte array=w366:u8[])
                n157 = String To Byte Array(string=w334) -> (unsigned byte array=w332:u8[])
                n158 = String To Byte Array(string=w339) -> (unsigned byte array=w338:u8[])
                n159 = String To Byte Array(string=w355) -> (unsigned byte array=w359:u8[])
                n160 = String To Byte Array(string=w348) -> (unsigned byte array=w352:u8[])
                n161 = String To Byte Array(string=w341) -> (unsigned byte array=w345:u8[])
                n162 = Index Array(array=w332, index=0) -> (element=w333:u8)
                n163 = Index Array(array=w338, index=0) -> (element=w314:u8)
                n164 = Index Array(array=w366, index=1) -> (element=w364:u8)
                n165 = To Byte Integer(number=w333) -> (8bit integer=w313:i8)
                n166 = Index Array(array=w366, index=0) -> (element=w363:u8)
                n167 = Index Array(array=w359, index=1) -> (element=w357:u8)
                n168 = Index Array(array=w352, index=1) -> (element=w350:u8)
                n169 = Index Array(array=w345, index=1) -> (element=w343:u8)
                n170 = Index Array(array=w359, index=0) -> (element=w356:u8)
                n171 = Index Array(array=w352, index=0) -> (element=w349:u8)
                n172 = Index Array(array=w345, index=0) -> (element=w342:u8)
                n173 = Join Numbers(hi=w363, lo=w364) -> ((hi.lo)=w315:u16)
                n174 = Join Numbers(hi=w356, lo=w357) -> ((hi.lo)=w312:u16)
                n175 = Join Numbers(hi=w349, lo=w350) -> ((hi.lo)=w311:u16)
                n176 = Join Numbers(hi=w342, lo=w343) -> ((hi.lo)=w310:u16)
                n177 = Bundle(w315, w314, w313, w312, w311, w310) -> (w309:cluster{u16, u8, i8, u16, u16, u16})  [unwired: 1 in]
              }
              n178 = Bundle("data"=w302, w300) -> (w299:T7)  [unwired: 1 in]
            }
            frame 130 {
              n179 = String Subset(string=w373, offset (0)=11, length (rest)=1 ("length (rest)")) -> (substring=w382:string)
              n180 = String Subset(string=w373, offset (0)=12, length (rest)=1 ("length (rest)")) -> (substring=w377:string)
              n181 = String To Byte Array(string=w382) -> (unsigned byte array=w381:u8[])
              n182 = String To Byte Array(string=w377) -> (unsigned byte array=w376:u8[])
              n183 = Index Array(array=w381, index=0) -> (element=w371:u8)
              n184 = Index Array(array=w376, index=0) -> (element=w374:u8)
              n185 = for {
                N: w374 -> [_]
                tunnel: w373 -> [w393]
                tunnel: [w385] -> w370 mode=indexing
                i -> [w390]
                # "må endres til 2 comp for negative verdi"
                n186 = Multiply(x=w390, y=4) -> (x*y=w389:i32)
                n187 = Add(x=13 ("offset (0)"), y=w389) -> (x+y=w407:i32)
                n188 = Add(x=15 ("offset (0)"), y=w389) -> (x+y=w400:i32)
                n189 = Add(x=16 ("offset (0)"), y=w389) -> (x+y=w394:i32)
                n190 = String Subset(string=w393, offset (0)=w400, length (rest)=1 ("length (rest)")) -> (substring=w403:string)
                n191 = String Subset(string=w393, offset (0)=w407, length (rest)=2 ("length (rest)")) -> (substring=w408:string)
                n192 = String Subset(string=w393, offset (0)=w394, length (rest)=1 ("length (rest)")) -> (substring=w397:string)
                n193 = String To Byte Array(string=w403) -> (unsigned byte array=w401:u8[])
                n194 = String To Byte Array(string=w408) -> (unsigned byte array=w412:u8[])
                n195 = String To Byte Array(string=w397) -> (unsigned byte array=w396:u8[])
                n196 = Index Array(array=w401, index=0) -> (element=w402:u8)
                n197 = Index Array(array=w396, index=0) -> (element=w386:u8)
                n198 = To Byte Integer(number=w402) -> (8bit integer=w387:i8)
                n199 = Index Array(array=w412, index=1) -> (element=w410:u8)
                n200 = Index Array(array=w412, index=0) -> (element=w409:u8)
                n201 = Join Numbers(hi=w409, lo=w410) -> ((hi.lo)=w388:u16)
                n202 = Bundle(w388, w387, w386) -> (w385:cluster{u16, i8, u8})  [unwired: 1 in]
              }
              n203 = Bundle("data"=w372, w371, w370) -> (w369:T8)  [unwired: 1 in]
            }
          }
        }
      }
    }
    frame 23 {
      # "network time"
      n204 = String Subset(string=w418, offset (0)=17, length (rest)=5 ("length (rest)")) -> (substring=w421:string)
      n205 = String Subset(string=w418, offset (0)=22, length (rest)=2 ("length (rest)")) -> (substring=w430:string)
      n206 = String Subset(string=w418, offset (0)=1, length (rest)=4 ("length (rest)")) -> (substring=w433:string)
      n207 = String Subset(string=w418, offset (0)=13, length (rest)=4 ("length (rest)")) -> (substring=w431:string)
      n208 = String Subset(string=w418, offset (0)=5, length (rest)=8 ("length (rest)")) -> (substring=w432:string)
      n209 = Unflatten From String(type=u64 0 ("index"), binary string=w432) -> (value=w429:u64)  [unwired: 3 in, 2 out]
      n210 = Unflatten From String(type=u16 0 ("index"), binary string=w430) -> (value=w420:u16)  [unwired: 3 in, 2 out]
      n211 = Unflatten From String(type=u32 0 ("index"), binary string=w431) -> (value=w428:u32)  [unwired: 3 in, 2 out]
      n212 = Unflatten From String(type=u32 0 ("index"), binary string=w433) -> (value=w423:u32)  [unwired: 3 in, 2 out]
      n213 = call "smartmeshIP to ni timestamp.vi"("use correction"=w415, "set corr due to mismatch in manager time"=TRUE, "microeconds"=w428, "seconds"=w429) -> ("Dust Timestamp"=w422:timestamp)  [unwired: 7 in]
      n214 = Bundle("index"=w423, "Dust Timestamp"=w422, "data"=w421, "index"=w420) -> (w419:T4)  [unwired: 1 in]
    }
    frame 48 {
      # "getPathInfo"
      n215 = String Subset(string=w456, offset (0)=17, length (rest)=5 ("length (rest)")) -> (substring=w463:string)
      n216 = String Subset(string=w456, offset (0)=9, length (rest)=8 ("length (rest)")) -> (substring=w455:string)
      n217 = String Subset(string=w456, offset (0)=1, length (rest)=8 ("length (rest)")) -> (substring=w445:string)
      n218 = String To Byte Array(string=w463) -> (unsigned byte array=w459:u8[])
      n219 = Index Array(array=w459, index=i8 4) -> (element=w448:u8)
      n220 = Index Array(array=w459, index=i8 3) -> (element=w450:u8)
      n221 = Index Array(array=w459, index=1) -> (element=w453:u8)
      n222 = Index Array(array=w459, index=0) -> (element=w454:u8)
      n223 = Index Array(array=w459, index=2) -> (element=w452:u8)
      n224 = To Byte Integer(number=w450) -> (8bit integer=w449:i8)
      n225 = To Byte Integer(number=w448) -> (8bit integer=w447:i8)
      n226 = Bundle("(hi.lo)"=u16 0, "data"=w445, "data"=w455, w454, w453, w452, w449, w447) -> (w451:T9)  [unwired: 1 in]
    }
    frame 49 {
      # "getNextPath"
      n227 = String Subset(string=w487, offset (0)=19, length (rest)=5 ("length (rest)")) -> (substring=w497:string)
      n228 = String Subset(string=w487, offset (0)=11, length (rest)=8 ("length (rest)")) -> (substring=w471:string)
      n229 = String Subset(string=w487, offset (0)=3, length (rest)=8 ("length (rest)")) -> (substring=w472:string)
      n230 = String Subset(string=w487, offset (0)=1, length (rest)=2 ("length (rest)")) -> (substring=w488:string)
      n231 = String To Byte Array(string=w497) -> (unsigned byte array=w493:u8[])
      n232 = String To Byte Array(string=w488) -> (unsigned byte array=w476:u8[])
      n233 = Index Array(array=w493, index=i8 4) -> (element=w479:u8)
      n234 = Index Array(array=w493, index=i8 3) -> (element=w481:u8)
      n235 = Index Array(array=w493, index=1) -> (element=w485:u8)
      n236 = Index Array(array=w493, index=0) -> (element=w486:u8)
      n237 = Index Array(array=w493, index=2) -> (element=w484:u8)
      n238 = Index Array(array=w476, index=0) -> (element=w475:u8)
      n239 = To Byte Integer(number=w481) -> (8bit integer=w480:i8)
      n240 = To Byte Integer(number=w479) -> (8bit integer=w478:i8)
      n241 = Index Array(array=w476, index=1) -> (element=w474:u8)
      n242 = Join Numbers(hi=w475, lo=w474) -> ((hi.lo)=w473:u16)
      n243 = Bundle(w473, "data"=w472, "data"=w471, w486, w485, w484, w480, w478) -> (w483:T10)  [unwired: 1 in]
    }
    frame 62 {
      # "getMoteInfo"
      n244 = String Subset(string=w517, offset (0)=9, length (rest)=27 ("length (rest)")) -> (substring=w561:string)
      n245 = String Subset(string=w517, offset (0)=1, length (rest)=8 ("length (rest)")) -> (substring=w505:string)
      n246 = String To Byte Array(string=w561) -> (unsigned byte array=w516:u8[])
      n247 = Index Array(array=w516, index=4) -> (element=w579:u8)
      n248 = Index Array(array=w516, index=1) -> (element=w514:u8)
      n249 = Index Array(array=w516, index=6) -> (element=w575:u8)
      n250 = Index Array(array=w516, index=8) -> (element=w569:u8)
      n251 = Index Array(array=w516, index=10) -> (element=w565:u8)
      n252 = Index Array(array=w516, index=0) -> (element=w515:u8)
      n253 = Index Array(array=w516, index=2) -> (element=w513:u8)
      n254 = Index Array(array=w516, index=3) -> (element=w578:u8)
      n255 = Index Array(array=w516, index=5) -> (element=w574:u8)
      n256 = Index Array(array=w516, index=7) -> (element=w568:u8)
      n257 = Index Array(array=w516, index=9) -> (element=w564:u8)
      n258 = Join Numbers(hi=w578, lo=w579) -> ((hi.lo)=w572:u16)
      n259 = Join Numbers(hi=w574, lo=w575) -> ((hi.lo)=w573:u16)
      n260 = Join Numbers(hi=w568, lo=w569) -> ((hi.lo)=w562:u16)
      n261 = Join Numbers(hi=w564, lo=w565) -> ((hi.lo)=w563:u16)
      n262 = Join Numbers(hi=w572, lo=w573) -> ((hi.lo)=w512:u32)
      n263 = Join Numbers(hi=w562, lo=w563) -> ((hi.lo)=w511:u32)
      n264 = Index Array(array=w516, index=12) -> (element=w558:u8)
      n265 = Index Array(array=w516, index=14) -> (element=w554:u8)
      n266 = Index Array(array=w516, index=16) -> (element=w548:u8)
      n267 = Index Array(array=w516, index=18) -> (element=w544:u8)
      n268 = Index Array(array=w516, index=11) -> (element=w557:u8)
      n269 = Index Array(array=w516, index=13) -> (element=w553:u8)
      n270 = Index Array(array=w516, index=15) -> (element=w547:u8)
      n271 = Index Array(array=w516, index=17) -> (element=w543:u8)
      n272 = Join Numbers(hi=w557, lo=w558) -> ((hi.lo)=w551:u16)
      n273 = Join Numbers(hi=w553, lo=w554) -> ((hi.lo)=w552:u16)
      n274 = Join Numbers(hi=w547, lo=w548) -> ((hi.lo)=w541:u16)
      n275 = Join Numbers(hi=w543, lo=w544) -> ((hi.lo)=w542:u16)
      n276 = Join Numbers(hi=w551, lo=w552) -> ((hi.lo)=w510:u32)
      n277 = Join Numbers(hi=w541, lo=w542) -> ((hi.lo)=w509:u32)
      n278 = Index Array(array=w516, index=20) -> (element=w538:u8)
      n279 = Index Array(array=w516, index=22) -> (element=w534:u8)
      n280 = Index Array(array=w516, index=24) -> (element=w528:u8)
      n281 = Index Array(array=w516, index=26) -> (element=w524:u8)
      n282 = Index Array(array=w516, index=19) -> (element=w537:u8)
      n283 = Index Array(array=w516, index=21) -> (element=w533:u8)
      n284 = Index Array(array=w516, index=23) -> (element=w527:u8)
      n285 = Index Array(array=w516, index=25) -> (element=w523:u8)
      n286 = Join Numbers(hi=w537, lo=w538) -> ((hi.lo)=w531:u16)
      n287 = Join Numbers(hi=w533, lo=w534) -> ((hi.lo)=w532:u16)
      n288 = Join Numbers(hi=w527, lo=w528) -> ((hi.lo)=w521:u16)
      n289 = Join Numbers(hi=w523, lo=w524) -> ((hi.lo)=w522:u16)
      n290 = Join Numbers(hi=w531, lo=w532) -> ((hi.lo)=w508:u32)
      n291 = Join Numbers(hi=w521, lo=w522) -> ((hi.lo)=w507:u32)
      n292 = Bundle("data"=w505, w515, w514, w513, w512, w511, w510, w509, w508, w507) -> (w506:T11)  [unwired: 1 in]
    }
    frame 47 {
      # "getMoteConfig"
      n293 = String Subset(string=w599, offset (0)=9, length (rest)=27 ("length (rest)")) -> (substring=w603:string)
      n294 = String Subset(string=w599, offset (0)=1, length (rest)=8 ("length (rest)")) -> (substring=w597:string)
      n295 = String To Byte Array(string=w603) -> (unsigned byte array=w598:u8[])
      n296 = Index Array(array=w598, index=4) -> (element=w593:u8)
      n297 = Index Array(array=w598, index=1) -> (element=w596:u8)
      n298 = Index Array(array=w598, index=0) -> (element=w595:u8)
      n299 = Index Array(array=w598, index=2) -> (element=w591:u8)
      n300 = Index Array(array=w598, index=3) -> (element=w592:u8)
      n301 = Index Array(array=w598, index=5) -> (element=w589:u8)
      n302 = Join Numbers(hi=w595, lo=w596) -> ((hi.lo)=w594:u16)
      n303 = Greater Than 0?(x=w591) -> (x > 0?=w590:bool)
      n304 = Greater Than 0?(x=w589) -> (x > 0?=w588:bool)
      n305 = Bundle("data"=w597, w594, w590, w592, w593, w588) -> (w587:cluster{"data":string, u16, bool, u8, u8, bool})  [unwired: 1 in]
    }
    frame 65 {
      # "getMoteConfigByID"
      n306 = String Subset(string=w624, offset (0)=9, length (rest)=27 ("length (rest)")) -> (substring=w628:string)
      n307 = String Subset(string=w624, offset (0)=1, length (rest)=8 ("length (rest)")) -> (substring=w622:string)
      n308 = String To Byte Array(string=w628) -> (unsigned byte array=w623:u8[])
      n309 = Index Array(array=w623, index=4) -> (element=w618:u8)
      n310 = Index Array(array=w623, index=1) -> (element=w621:u8)
      n311 = Index Array(array=w623, index=0) -> (element=w620:u8)
      n312 = Index Array(array=w623, index=2) -> (element=w616:u8)
      n313 = Index Array(array=w623, index=3) -> (element=w617:u8)
      n314 = Index Array(array=w623, index=5) -> (element=w614:u8)
      n315 = Join Numbers(hi=w620, lo=w621) -> ((hi.lo)=w619:u16)
      n316 = Greater Than 0?(x=w616) -> (x > 0?=w615:bool)
      n317 = Greater Than 0?(x=w614) -> (x > 0?=w613:bool)
      n318 = Bundle("data"=w622, w619, w615, w617, w618, w613) -> (w612:cluster{"data":string, u16, bool, u8, u8, bool})  [unwired: 1 in]
    }
  }
  "Data Notifications" <- w13
  "network time" <- w5
  "error out" <- w3
  n319 = Bundle(w12, w10, w11, w9, w8, w7, w4) -> (→"mote and link status":T12)  [unwired: 1 in]
